vi "SUMM-2bit.vi"(2 "b0":bool, 3 "a0":bool, 4 "OP":bool) -> (0 "S0":bool, 1 "S1":bool)   [LabVIEW 2012]
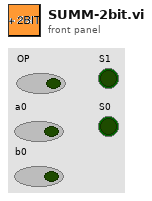
[diagram p1: front panel]
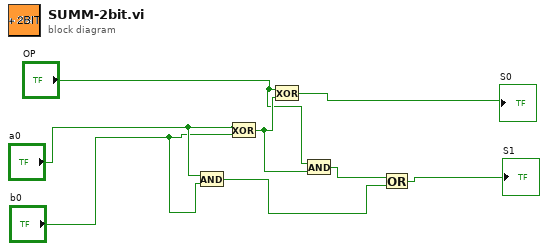
[diagram p0: block diagram]
diagram:
  n1 = And(x="a0", y="b0") -> (x .and. y?=w8:bool)
  n2 = Exclusive Or(1:"b0", 2:"a0") -> (0:w7:bool)
  n3 = Exclusive Or(1:w7, 2:"OP") -> (0:→"S0":bool)
  n4 = And(x="OP", y=w7) -> (x .and. y?=w6:bool)
  n5 = Or(x=w6, y=w8) -> (x .or. y?=→"S1":bool)
